vi "ukol 1.vi"() -> ()   [LabVIEW 2023]
uses:
  <vilib>/measure/maspectr.llb/Power Spectrum and PSD Export Mode.ctl
  <vilib>/measure/maspectr.llb/FFT Power Spectrum and PSD for 1 Chan.vi
  <vilib>/measure/NI_MABase.lvlib
  <vilib>/measure/NI_MAPro.lvlib
  <vilib>/Analysis/NI_AALBase.lvlib
panel:
  out "Histogram Graph":T1(graph)
  out "spektrum":cluster{"f0":dbl, "df":dbl, "magnitude":dbl[]}[](graph)
  out "Waveform Graph":waveform(dbl)[](graph)
  in  "sampling info":cluster{"Fs":dbl, "#s":dbl}={"Fs"=1000.0, "#s"=1000.0} {"Fs" format="%.2p"}
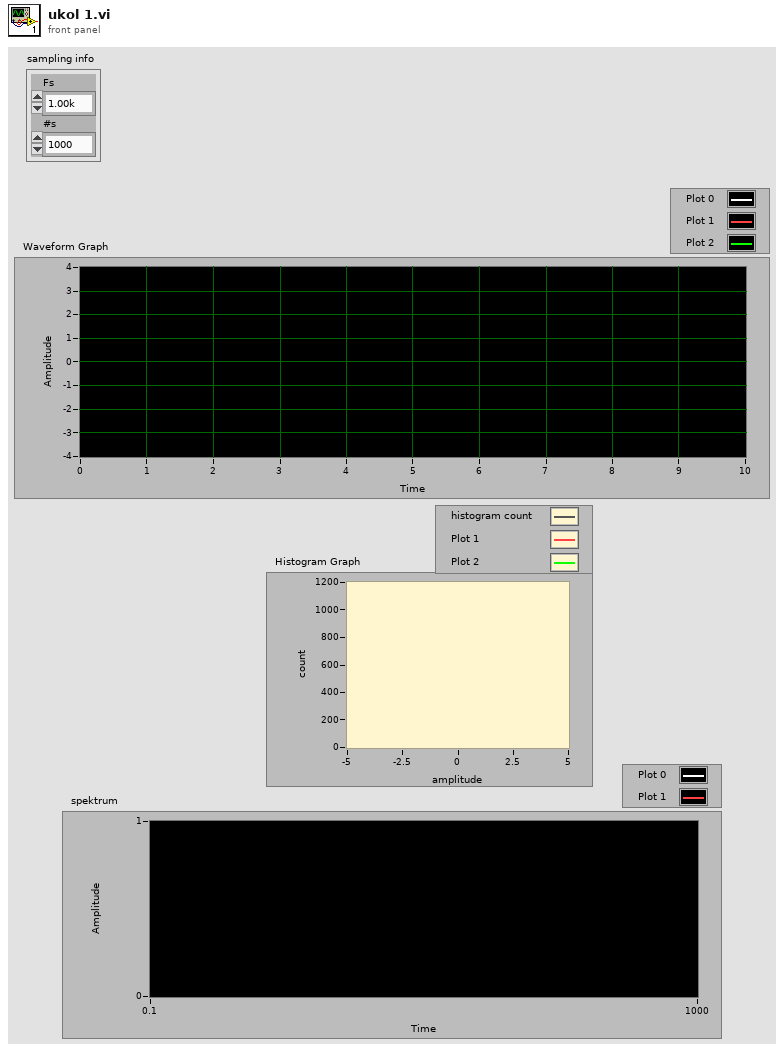
[diagram p1: front panel]
types:
  T1 = cluster{"X Values":dbl[], "Histogram: h(x)":i32[]}[]
  T2 = typedef "NI_MAPro.lvlib/Power Spectrum and PSD Export Mode.ctl" = u16
  T3 = cluster{"X Values":dbl[], "Histogram: h(x)":i32[]}
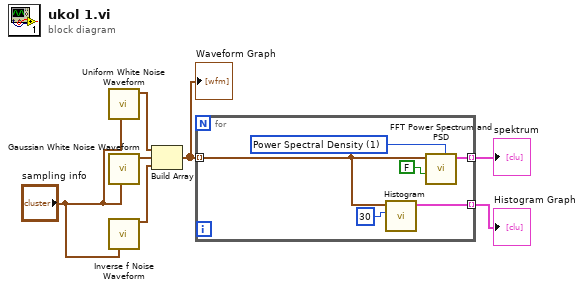
[diagram p0: block diagram]
diagram:
  n1 = call <vilib>:"Uniform White Noise Waveform.vi"("sampling info"="sampling info") -> ("signal out"=w6:waveform(dbl))  [unwired: 9 in, 1 out]
  n2 = call <vilib>:"Gaussian White Noise Waveform.vi"("sampling info"="sampling info") -> ("signal out"=w5:waveform(dbl))  [unwired: 9 in, 1 out]
  n3 = call <vilib>:"Inverse f Noise Waveform.vi"("sampling info"="sampling info") -> ("signal out"=w4:waveform(dbl))  [unwired: 10 in, 4 out]
  n4 = Build Array(w6, w5, w4) -> (w3:waveform(dbl)[])
  "Waveform Graph" <- w3
  n5 = for {
    tunnel: w3 -> [w8] mode=indexing
    tunnel: [w10] -> w2 mode=indexing
    tunnel: [w9] -> w1 mode=indexing
    w13 = T2 1 items=["Power Spectrum", "Power Spectral Density"] ("export mode")
    n6 = call <vilib>:"Histogram.vi"("intervals"=30, "X"=w8) -> ("Histogram Graph"=w9:T3)  [unwired: 6 in, 3 out]
    n7 = call-poly <vilib>:"FFT Power Spectrum and PSD.vi"("export mode"=w13, "dB On (F)"=FALSE, "time signal"=w8) -> ("Power Spectrum / PSD"=w10:cluster{"f0":dbl, "df":dbl, "magnitude":dbl[]})  [unwired: 5 in, 3 out]
  }
  "spektrum" <- w2
  "Histogram Graph" <- w1
